vi "Load Overlay.vi"(8 "error in (no error)":errorcluster, 10 "Config":refnum<class "Config Manager.lvclass">, 11 "Config Storage in":refnum<class "Config Storage.lvclass">) -> (0 "error out":errorcluster, 3 "Config Storage out":refnum<class "Config Storage.lvclass">)   [LabVIEW 2023, in "CDM-Config.lvlib" / "Config Storage.lvclass"]
doc: "Loads a filtered saved config into an existing config. This uses the <b>Set Root Element</b> value (alternatively set via <b>Set Root Hierarchy</b>) set on the storage instance for reloading subtrees so ensure that has been specified if necessary.\n\nOverlays are partial configs that either limit to a subtree of a full config or to specific meta values. When loading an overlay, values and meta fields are overwritten with values from the saved overlay."
uses:
  Config Storage.lvclass
  Config Manager/Config Manager.lvclass
  Config Storage.lvclass/Config Storage.ctl
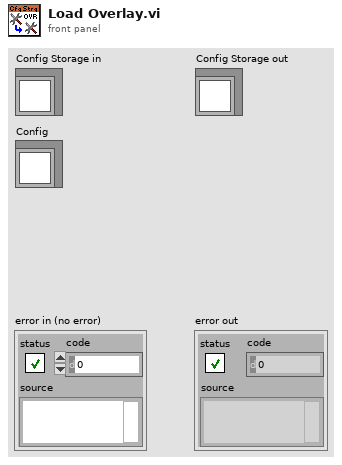
[diagram p1: front panel]
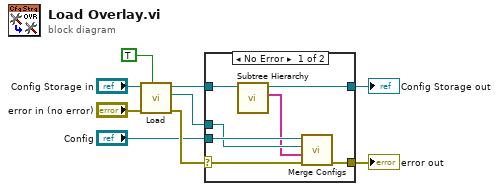
[diagram p0: block diagram]
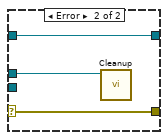
[diagram p2: hidden frame]
diagram:
  n1 = call "Load.vi"("Mutable (F)"=TRUE, "error in (no error)"="error in (no error)", "Config Storage in"="Config Storage in") -> ("error out"=w6:errorcluster, "Config"=w3:refnum<class "Config Manager.lvclass">, "Config Storage out"=w5:refnum<class "Config Storage.lvclass">)  [unwired: 6 in]
  n2 = case shown="No Error" w6 {
    selector: w6 -> [w14 w18]
    tunnel: "Config" -> [w16 _]
    tunnel: w3 -> [w15 w19]
    tunnel: [w13 w18] -> w7
    tunnel: w5 -> [w12 w17]
    tunnel: [w11 w17] -> w2
    frame No Error {
      n3 = call "Subtree Hierarchy.vi"("Config Storage in"=w12) -> ("Subtree Hierarchy"=w10:string[], "Config Storage out"=w11:refnum<class "Config Storage.lvclass">)  [unwired: 8 in, 1 out]
      n4 = call "Merge Configs.vi"("error in (no error)"=w14, "Merge Hierarchy (Root)"=w10, "From Config"=w15, "Config Manager in"=w16) -> ("error out"=w13:errorcluster)  [unwired: 6 in, 1 out]
    }
    frame Error {
      n5 = call "Cleanup.vi"("Config Manager in"=w19) -> ()  [unwired: 10 in, 1 out]
    }
  }
  "error out" <- w7
  "Config Storage out" <- w2
